vi "EditOptions.vi"(8 "error in":errorcluster, 11 "HW Engine in":refnum<class "HW Engine.lvclass">) -> (0 "error out":errorcluster, 1 "edit options":T1, 2 "subnodes class":T2, 3 "HW Engine out":refnum<class "HW Engine.lvclass">)   [LabVIEW 2025, in "HW Engine.lvlib" / "HW Engine.lvclass"]
doc: "This VI Contains the options for the Menu that will be displayed when doing right click on an item\nThe subnodes class configures which nodes can be added to this nodes\nAnd the edit options determine which options are available for the node.\n\nThis configuration is stored in this VI in case some dynamic configuration is required for the menu options or subnodes.\n\nAll VIs must overide this methodCopyright 2017 National Instruments Corporation\n\nLicensed under the Apache License, Version 2.0 (the \"License\"); you may not use this file except in compliance with the License. You may obtain a copy of the License at http://www.apache.org/licenses/LICENSE-2.0\nUnless required by applicable law or agreed to in writing, software distributed under the License is distributed on an \"AS IS\" BASIS, WITHOUT WARRANTIES OR CONDITIONS OF ANY KIND, either express or implied. See the License for the specific language governing permissions and limitations under the License."
uses:
  HW Engine.lvclass
  Users/Public/Documents/Sandia National Labs/TSS Plugin/CEF.lvlibp/Node/SubNodeCluster.ctl
  Users/Public/Documents/Sandia National Labs/TSS Plugin/CEF.lvlibp/Node/NodeMenuOptions.ctl
  HW Engine.lvclass/HW Engine.ctl
  Users/Public/Documents/Sandia National Labs/TSS Plugin/CEF.lvlibp/Node/CEF_Node.lvclass
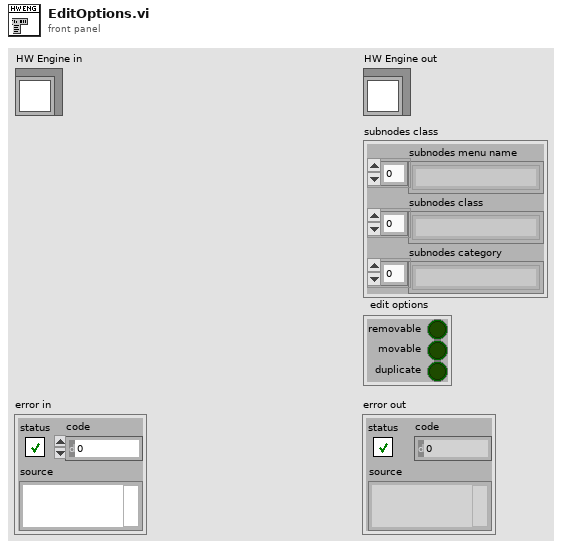
[diagram p1: front panel]
types:
  T1 = typedef "CEF.lvlibp/CEF_Node.lvclass/NodeMenuOptions.ctl" = cluster{"removable":bool, "movable":bool, "duplicate":bool}
  T2 = typedef "CEF.lvlibp/CEF_Node.lvclass/SubNodeCluster.ctl" = cluster{"subnodes menu name":string[], "subnodes class":string[], "subnodes category":string[]}
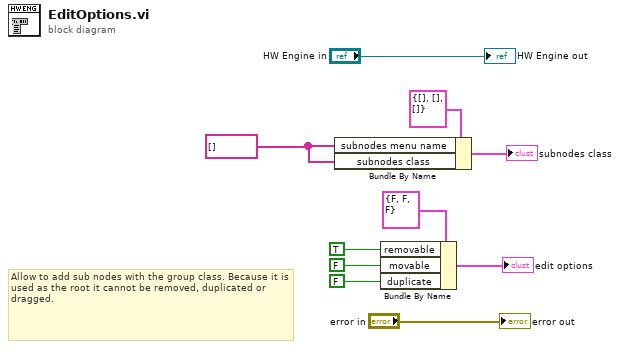
[diagram p0: block diagram]
diagram:
  w1 = string[] [] ("subnodes menu name")
  # "Allow to add sub nodes with the group class. Because it is used as the root it cannot be removed, duplicated or dragged."
  n1 = Bundle By Name(cluster=T2 {"subnodes menu name"=[], "subnodes class"=[], "subnodes category"=[]} ("subnodes class"), "subnodes menu name"=w1, "subnodes class"=w1) -> (→"subnodes class":T2)
  n2 = Bundle By Name(cluster=T1 {"removable"=FALSE, "movable"=FALSE, "duplicate"=FALSE} ("edit options"), "removable"=TRUE ("Removable"), "movable"=FALSE ("Movable"), "duplicate"=FALSE ("Duplicate")) -> (→"edit options":T1)
  "error out" <- "error in"
  "HW Engine out" <- "HW Engine in"
